vi "Generate SOQPSK Filter Coefficients.vi"(8 "error in":errorcluster) -> (0 "error out":errorcluster, 1 "filter length (samples)":u16, 2 "matched filter coefficients":dbl[](array[numeric]), 3 "symmetric filter coefficients":T1, 4 "samples per bit":u16)   [LabVIEW 2023, in "SOQPSK Host Support.lvlib"]
uses:
  SOQPSK Host Support.lvlib
  <vilib>/addons/Modulation/Analog/support/mod_Set Error Source.vi
  <vilib>/addons/Modulation/Digital/Support/Common/Validators/mod_Generate Filter Coefficients Validate.vi
  <vilib>/addons/Modulation/Digital/General/subVIs/mod_Generate Filter Coefficients.vi
  <vilib>/addons/Modulation/niDMT.lvlib
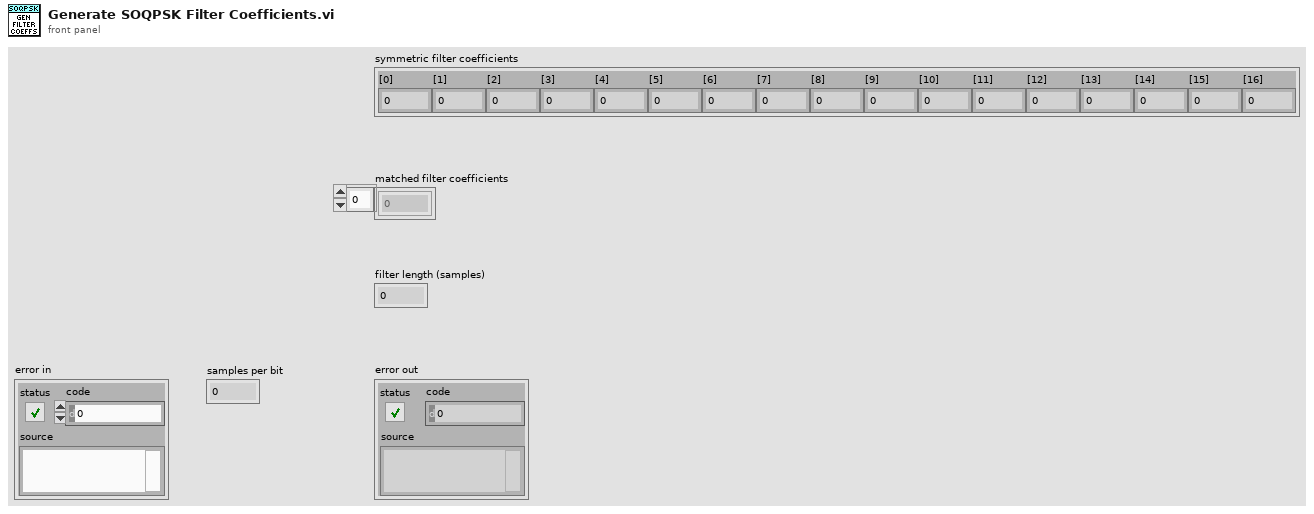
[diagram p1: front panel]
types:
  T1 = cluster{"[0]":fxp<+/-,16,1>, "[1]":fxp<+/-,16,1>, "[2]":fxp<+/-,16,1>, "[3]":fxp<+/-,16,1>, "[4]":fxp<+/-,16,1>, "[5]":fxp<+/-,16,1>, "[6]":fxp<+/-,16,1>, "[7]":fxp<+/-,16,1>, "[8]":fxp<+/-,16,1>, "[9]":fxp<+/-,16,1>, "[10]":fxp<+/-,16,1>, "[11]":fxp<+/-,16,1>, "[12]":fxp<+/-,16,1>, "[13]":fxp<+/-,16,1>, "[14]":fxp<+/-,16,1>, "[15]":fxp<+/-,16,1>, "[16]":fxp<+/-,16,1>}
  T2 = cluster{"TX Filter":enum16{"none", "Raised Cosine", "Root Raised Cos", "Gaussian"}, "Alpha":dbl, "Filter Length (symbols)":i32}
  T3 = enum16{"FSK", "PSK", "QAM", "MSK", "PAM", "ASK", "CPM"}
  T4 = enum16{"none", "Raised Cosine", "Root Raised Cos", "Gaussian"}
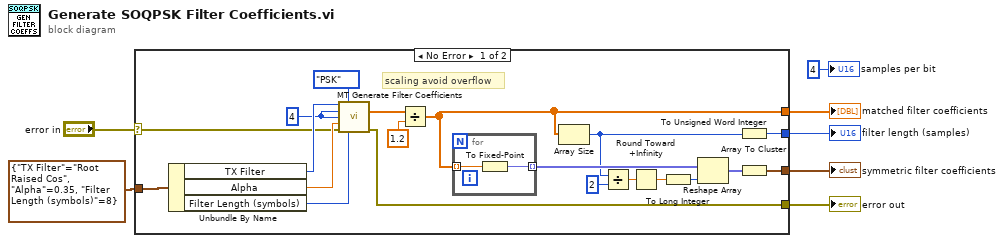
[diagram p0: block diagram]
diagram:
  n1 = case shown="No Error" "error in" {
    selector: "error in" -> [w19 w30]
    tunnel: [w9 _] -> w7
    tunnel: [w26 _] -> w6
    tunnel: [w25 _] -> w3
    tunnel: T2 {"TX Filter"=enum."Root Raised Cos", "Alpha"=0.35, "Filter Length (symbols)"=8} ("Filter Parameters") -> [w21 _]
    tunnel: [w18 w30] -> w4
    frame No Error {
      w11 = 4 ("matched samples per symbol (16)")
      # "scaling avoid overflow"
      n2 = Unbundle By Name(w21) -> ("TX Filter"=w22:T4, "Alpha"=w23:dbl, "Filter Length (symbols)"=w24:i32)
      n3 = call <vilib>:"MT Generate Filter Coefficients.vi"("pulse shaping filter (none)"=w22, "modulation type"=T3."PSK", "pulse shaping samples per symbol (16)"=w11, "matched samples per symbol (16)"=w11, "filter parameter"=w23, "error in (no error)"=w19, "filter length (symbols)"=w24) -> ("matched filter coefficients"=w10:dbl[], "error out"=w18:errorcluster)  [unwired: 6 in, 1 out]
      n4 = Divide(x=w10, y=1.2) -> (x/y=w9:dbl[])
      n5 = for {
        tunnel: w9 -> [w29] mode=indexing
        tunnel: [w28] -> w17 mode=indexing
        n6 = To Fixed-Point(number=w29) -> (fixed-point=w28:fxp<+/-,16,1>)  [unwired: 1 in]
      }
      n7 = Array Size(array=w9) -> (size(s)=w16:i32)
      n8 = Divide(x=w16, y=2) -> (x/y=w14:dbl)
      n9 = Round Toward +Infinity(x=w14) -> (ceil(x): smallest int >= x=w13:dbl)
      n10 = To Long Integer(number=w13) -> (32bit integer=w12:i32)
      n11 = Reshape Array(w17, w12) -> (w27:fxp<+/-,16,1>[])
      n12 = To Unsigned Word Integer(number=w16) -> (unsigned 16bit integer=w26:u16)
      n13 = Array To Cluster(array=w27) -> (cluster=w25:T1)
    }
    frame Error {
    }
  }
  "matched filter coefficients" <- w7
  "filter length (samples)" <- w6
  "error out" <- w4
  "symmetric filter coefficients" <- w3
  "samples per bit" <- u16 4 ("samples per bit")
